vi "Get Attribute as JSON.vi"(8 "error in":errorcluster, 10 "Attribute":string, 11 "Config from JSON in":refnum<class "Config from JSON.lvclass">) -> (0 "error out":errorcluster, 2 "<JSON>":string, 3 "Config from JSON out":refnum<class "Config from JSON.lvclass">)   [LabVIEW 2025, in "Config from JSON.lvclass"]
uses:
  Config from JSON.lvclass
  <vilib>/JDP Science/JSONtext/Next JSON Value.vi
  <vilib>/JDP Science/JSONtext/String Subset.vi
  <vilib>/JDP Science/JSONtext/Parsing/Advance past next JSON Value (inlined COPY).vi
  <vilib>/JDP Science/JSONtext/Parsing/Advance past whitespace.vi
  <vilib>/JDP Science/JSONtext/Parsing/Advance past String.vi
  <vilib>/JDP Science/JSONtext/Parsing/Advance past Number.vi
  <vilib>/JDP Science/JSONtext/Parsing/Advance past Line Ending.vi
  <vilib>/JDP Science/JSONtext/Parsing/Parse Full Path or Item Name.vi
  <vilib>/JDP Science/JSONtext/Parsing/Advance past Array.vi
  <vilib>/JDP Science/JSONtext/Parsing/Advance past Object.vi
  <vilib>/JDP Science/JSONtext/support/Error Cluster From Code.vi
  <vilib>/JDP Science/JSONtext/Offset/Find Item Locations by Path.vi
  <vilib>/JDP Science/JSONtext/JSONtext.lvlib
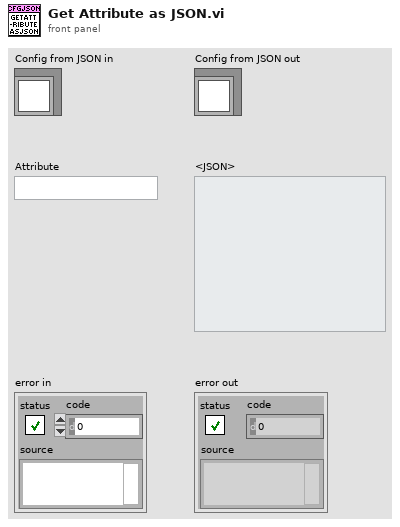
[diagram p1: front panel]
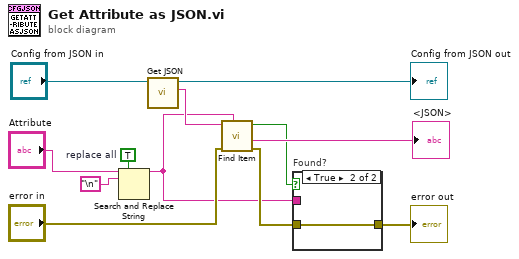
[diagram p0: block diagram]
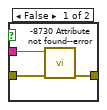
[diagram p2: hidden frame]
diagram:
  w3 = TRUE  # replace all
  n1 = Search and Replace String(replace all?=w3, input string="Attribute", search string="\n") -> (result string=w1:string)  [unwired: 5 in, 3 out]
  n2 = call-dynamic "Get JSON.vi"("ConfigFromJSON in"="Config from JSON in") -> ("<JSON>"=w10:string, "ConfigFromJSON out"=→"Config from JSON out":refnum<class "Config from JSON.lvclass">)  [unwired: 9 in]
  n3 = call <vilib>:"Find Item.vi"("$Path or Item Name"=w1, "error in (no error)"="error in", "JSON"=w10) -> ("error out"=w8:errorcluster, "<JSON>"=→"<JSON>":string, "Found"=w5:bool)  [unwired: 5 in, 1 out]
  n4 = case "Found?" shown="True" w5 {
    tunnel: w8 -> [w15 w16]
    tunnel: [w14 w16] -> w6
    tunnel: w1 -> [w13 _]
    frame False {
      n5 = call "-8730 Attribute not found--error.vi"("error in"=w15, "Attribute"=w13) -> ("error out"=w14:errorcluster)  [unwired: 9 in]
    }
    frame True {
    }
  }
  "error out" <- w6
